vi "set_imageType.vi"(8 "error in (no error)":errorcluster, 10 "Image Type":T1 items=["Grayscale (U8)", "Grayscale (I16)", "Grayscale (SGL)", "Complex (CSG)", "RGB (U32)", "HSL (U32)", "RGB (U64)", "Grayscale (U16)"], 11 "HGF_IMAQDevice":refnum<class "HGF_IMAQDevice.lvclass">) -> (0 "error out":errorcluster, 3 "HGF_IMAQDevice":refnum<class "HGF_IMAQDevice.lvclass">)   [LabVIEW 2014, in "HGF_IMAQ.lvlib" / "HGF_IMAQDevice.lvclass"]
uses:
  HGF_IMAQDevice.lvclass
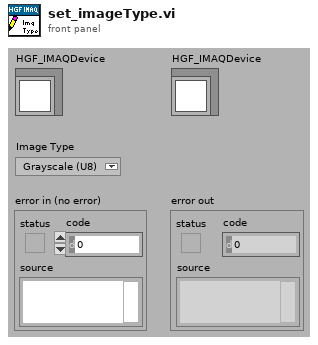
[diagram p1: front panel]
types:
  T1 = typedef "Image Type" = u32
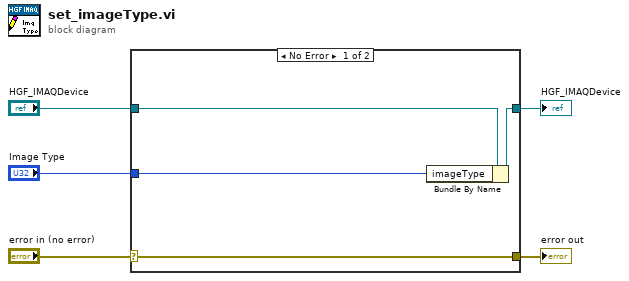
[diagram p0: block diagram]
diagram:
  n1 = case shown="No Error" "error in (no error)" {
    selector: "error in (no error)" -> [w9 w10]
    tunnel: [w9 w10] -> w4
    tunnel: [w7 w11] -> w2
    tunnel: "HGF_IMAQDevice" -> [w8 w11]
    tunnel: "Image Type" -> [w6 _]
    frame No Error {
      n2 = Bundle By Name(cluster=w8, "imageType"=w6) -> (w7:refnum<class "HGF_IMAQDevice.lvclass">)
    }
    frame Error {
    }
  }
  "error out" <- w4
  "HGF_IMAQDevice" <- w2
